vi "FindMatchingControls.vi"(4 "error in":errorcluster, 7 "Diagram":refnum<vi>) -> (0 "error out":errorcluster, 2 "MatchedControls":cluster{refnum<vi>, refnum<vi>}[](array[cluster]), 3 "Diagram out":refnum<vi>)   [LabVIEW 2017]
panel:
  # "LVHDF5 Toolkit\nCopyright (c) 2005-2013 by Jason D. Sommerville\nCopyright (c) 2014 by UPVI, LLC.\n\nThis use and distribution of this file is governed by the terms found in \nLICENSE.txt distributed with this toolkit and installed at\n <user.lib>\\_lvhdf5\\LICENSE.txt"
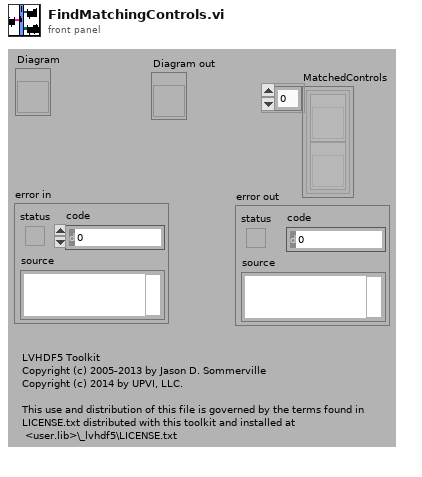
[diagram p1: front panel]
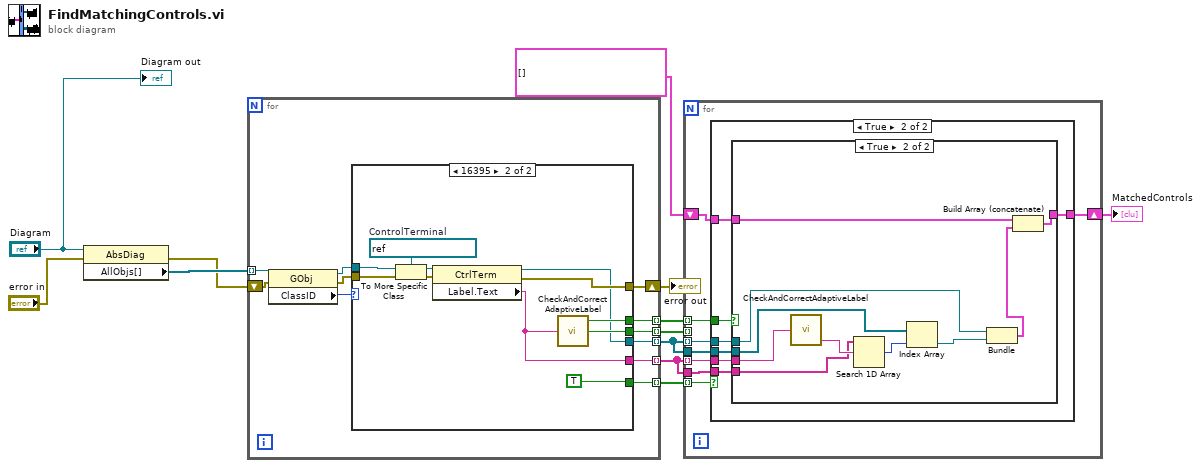
[diagram p0: block diagram]
diagram:
  n1 = property class="AbsDiag"(reference="Diagram", error in="error in") -> (error out=w9:errorcluster, "AllObjs[]"=w10:refnum<vi>[])  [unwired: 1 out]
  n2 = for {
    tunnel: w10 -> [w23] mode=indexing
    shift-right: [w15] -> w1
    shift-left: w9 -> [w19]
    tunnel: [w18] -> w5 mode=indexing
    tunnel: [w17] -> w7 mode=indexing
    tunnel: [w16] -> w6 mode=indexing
    tunnel: [w14] -> w8 mode=indexing
    tunnel: [w13] -> w4 mode=indexing
    n3 = property class="GObj"(reference=w23, error in=w19) -> (reference out=w20:refnum<vi>, error out=w21:errorcluster, "ClassID"=w22:u32)
    n4 = case shown="16395" w22 {
      tunnel: w21 -> [w24 w34]
      tunnel: w20 -> [_ w33]
      tunnel: [_ w27] -> w18
      tunnel: [_ w30] -> w17
      tunnel: [_ w29] -> w16
      tunnel: [w24 w28] -> w15
      tunnel: [_ TRUE] -> w14
      tunnel: [_ w25] -> w13
      frame 0, Default {
      }
      frame 16395 {
        w35 = refnum<vi> refnum  # ControlTerminal
        n5 = To More Specific Class(target class=w35, reference=w33, error in=w34) -> (specific class reference=w32:refnum<vi>, error out=w31:errorcluster)
        n6 = property class="CtrlTerm"(reference=w32, error in=w31) -> (reference out=w27:refnum<vi>, error out=w28:errorcluster, "Label.Text"=w25:string)
        n7 = call <vilib>:"CheckAndCorrectAdaptiveLabel.vi"("Control Label"=w25) -> ("Marked?"=w29:bool, "Adaptive?"=w30:bool)  [unwired: 1 out]
      }
    }
  }
  "error out" <- w1
  n8 = for {
    tunnel: w8 -> [w43] mode=indexing
    tunnel: w5 -> [w38] mode=indexing
    tunnel: w7 -> [_] mode=indexing
    tunnel: w6 -> [w42] mode=indexing
    tunnel: w4 -> [w41] mode=indexing
    tunnel: w5 -> [w39]
    tunnel: w4 -> [w40]
    shift-right: [w37] -> w2
    shift-left: cluster{refnum<vi>, refnum<vi>}[] [] -> [w36]
    n9 = case shown="True" w43 {
      tunnel: w42 -> [_ w51]
      tunnel: w41 -> [_ w50]
      tunnel: w40 -> [_ w49]
      tunnel: w39 -> [_ w48]
      tunnel: w38 -> [_ w47]
      tunnel: [w44 w46] -> w37
      tunnel: w36 -> [w44 w45]
      frame False {
      }
      frame True {
        n10 = case shown="True" w51 {
          tunnel: w50 -> [_ w62]
          tunnel: w49 -> [_ w60]
          tunnel: w48 -> [_ w58]
          tunnel: w47 -> [_ w56]
          tunnel: [w52 w54] -> w46
          tunnel: w45 -> [w52 w53]
          frame False {
          }
          frame True {
            n11 = call <vilib>:"CheckAndCorrectAdaptiveLabel.vi"("Control Label"=w62) -> ("Corrected Control Label"=w61:string)  [unwired: 2 out]
            n12 = Search 1D Array(1D array=w60, element=w61) -> (index of element=w59:i32)  [unwired: 1 in]
            n13 = Index Array(array=w58, index=w59) -> (element=w57:refnum<vi>)
            n14 = Bundle(w56, w57) -> (w55:cluster{refnum<vi>, refnum<vi>})  [unwired: 1 in]
            n15 = Build Array (concatenate)(w53, w55) -> (w54:cluster{refnum<vi>, refnum<vi>}[])
          }
        }
      }
    }
  }
  "MatchedControls" <- w2
  "Diagram out" <- "Diagram"
